vi "Initialize.vi"(8 "Error In":errorcluster, 11 "API Key":string) -> (0 "Error Out":errorcluster, 3 "Open Weather Session Out":refnum<class "Open Weather Session.lvclass">)   [LabVIEW 2019, in "Open Weather Session.lvclass"]
uses:
  Open Weather Session.lvclass
  Accessors/REST Client/Set REST Client.vi
  Accessors/API Key/Set API Key.vi
  <vilib>/addons/_JKI.lib/REST Client/classes/REST Client/REST Client.lvclass
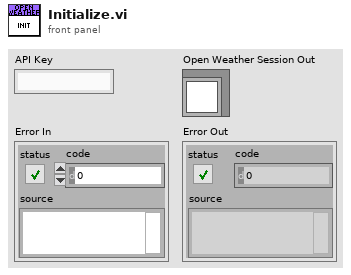
[diagram p1: front panel]
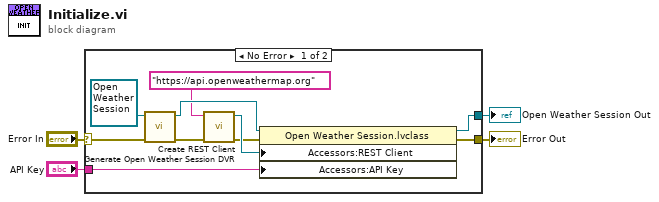
[diagram p0: block diagram]
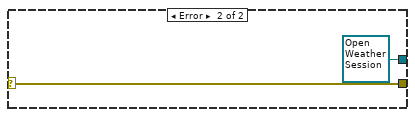
[diagram p2: hidden frame]
diagram:
  n1 = case shown="No Error" "Error In" {
    selector: "Error In" -> [w14 w16]
    tunnel: [w11 w16] -> w3
    tunnel: [w12 refnum<class "Open Weather Session.lvclass"> refnum ("Open Weather Session Out")] -> w2
    tunnel: "API Key" -> [w10 _]
    frame No Error {
      n2 = call "Generate Open Weather Session DVR.vi"("Error In"=w14, "Open Weather Session In"=refnum<class "Open Weather Session.lvclass"> refnum) -> ("Error Out"=w8:errorcluster, "Open Weather Session Out"=w13:refnum<class "Open Weather Session.lvclass">)  [unwired: 8 in]
      n3 = call <vilib>:"Create REST Client.vi"("error in (no error)"=w8, "Base URL"="https://api.openweathermap.org") -> ("error out"=w6:errorcluster, "REST Client out"=w7:refnum<class "REST Client.lvclass">)  [unwired: 8 in]
      n4 = property class="Open Weather Session.lvclass"(reference=w13, error in=w6, "Accessors:REST Client"=w7, "Accessors:API Key"=w10) -> (reference out=w12:refnum<class "Open Weather Session.lvclass">, error out=w11:errorcluster)
    }
    frame Error {
    }
  }
  "Open Weather Session Out" <- w2
  "Error Out" <- w3
